vi "写保持寄存器.vi"(7 "MB_实体":refnum<class "Modbus Master.lvclass">, 8 "error in":errorcluster, 11 "读保持寄存器信息组__输入":T1(array[cluster])) -> (0 "输出簇":errorcluster, 5 "连接成功":bool)   [LabVIEW 2015]
uses:
  <vilib>/NI/Modbus Library/API/Master/Modbus Master.lvclass
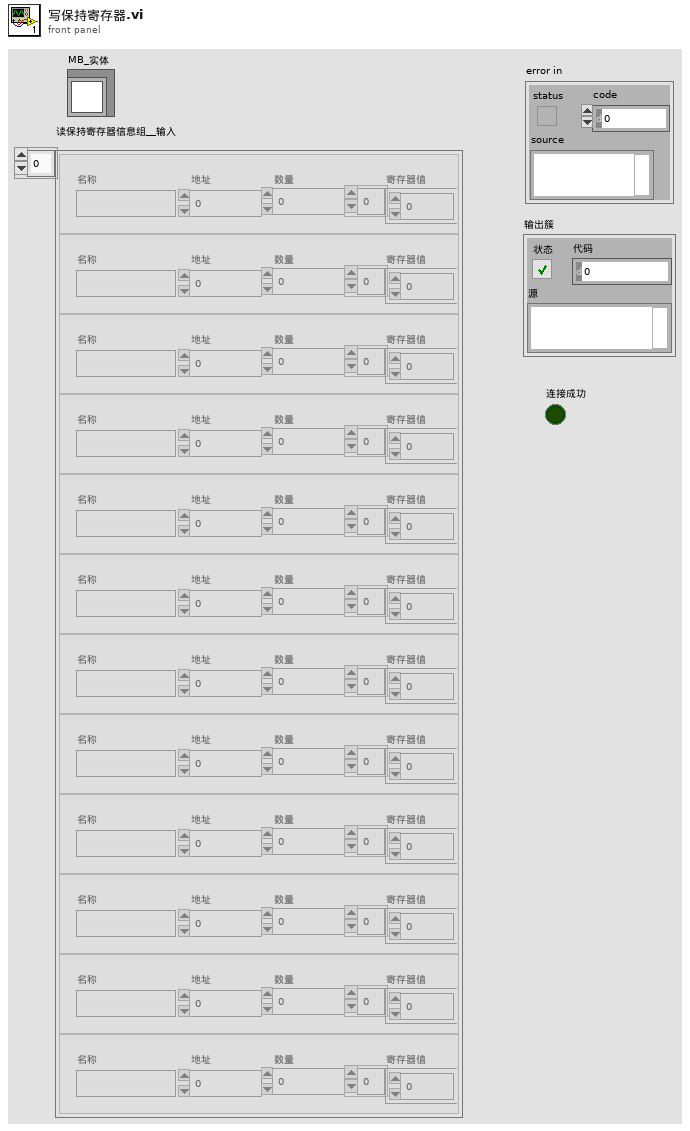
[diagram p1: front panel]
types:
  T1 = cluster{"地址":u16, "数量":u16, "寄存器值":u16[], "名称":string}[]
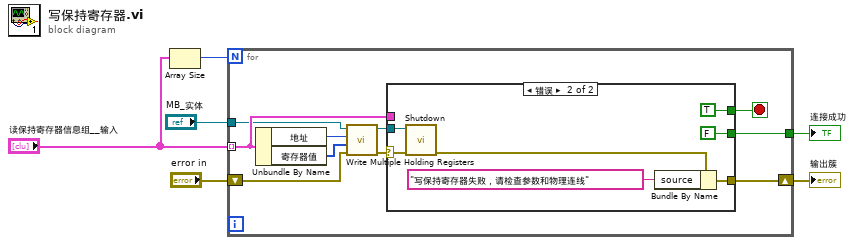
[diagram p0: block diagram]
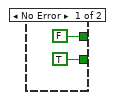
[diagram p2: hidden frame]
diagram:
  n1 = Array Size(array="读保持寄存器信息组__输入") -> (size(s)=w4:i32)
  n2 = for {
    N: w4 -> [_]
    tunnel: "读保持寄存器信息组__输入" -> [w15] mode=indexing
    tunnel: "MB_实体" -> [w12]
    shift-right: [w14] -> w2
    shift-left: "error in" -> [w10]
    tunnel: [w13] -> w1
    stop <- w16 stop-if-true
    n3 = Unbundle By Name(w15) -> ("地址"=w11:u16, "寄存器值"=w7:u16[])
    n4 = call-dynamic "Write Multiple Holding Registers.vi"("error in"=w10, "registers to write"=w7, "starting address"=w11, "Modbus master in"=w12) -> ("error out"=w9:errorcluster, "Modbus master out"=w8:refnum<class "Modbus Master.lvclass">)  [unwired: 6 in]
    n5 = case shown="错误" w9 {
      selector: w9 -> [_ w24]
      tunnel: w8 -> [_ w23]
      tunnel: [FALSE TRUE] -> w16
      tunnel: w15 -> [_ _]
      tunnel: [_ w21] -> w14
      tunnel: [TRUE FALSE] -> w13
      frame No Error {
      }
      frame Error {
        n6 = call-dynamic "Shutdown.vi"("error in"=w24, "Modbus master in"=w23) -> ("error out"=w22:errorcluster)  [unwired: 9 in]
        n7 = Bundle By Name(cluster=w22, "source"="写保持寄存器失败，请检查参数和物理连线" ("消息")) -> (w21:errorcluster)
      }
    }
  }
  "输出簇" <- w2
  "连接成功" <- w1
